vi "Point_Delete.vi"(8 "Error In":errorcluster, 10 "Tag":string, 11 "Map":T1) -> (0 "Error Out":errorcluster, 3 "Map Out":T1)   [LabVIEW 2017, in "PointValueMap.lvlib"]
doc: "Deletes a point from a map."
uses:
  <vilib>/addons/PointValueMap/PointValueMap.lvlib
  <vilib>/addons/PointValueMap/controls/PointMap.ctl
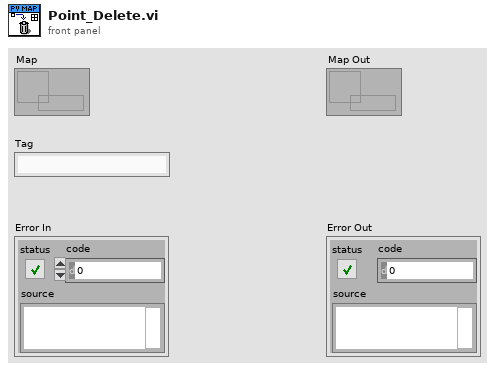
[diagram p1: front panel]
types:
  T1 = typedef "PointValueMap.lvlib/PointMap.ctl" = refnum<data-value>
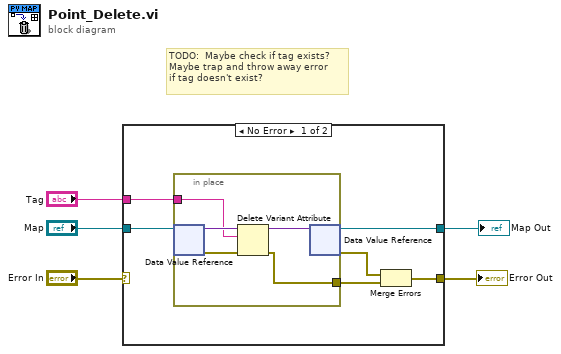
[diagram p0: block diagram]
diagram:
  # "TODO:  Maybe check if tag exists?\nMaybe trap and throw away error\nif tag doesn't exist?"
  n1 = case shown="No Error" "Error In" {
    selector: "Error In" -> [_ w18]
    tunnel: "Map" -> [w11 w17]
    tunnel: "Tag" -> [w10 _]
    tunnel: [w7 w18] -> w4
    tunnel: [w6 w17] -> w1
    frame No Error {
      n2 = in-place {
        in-place-border: w10 -> [w14]
        in-place-border: [w12] -> w8
        n3 = in-place-dvr #1(w11) -> (w16:variant, w15:errorcluster)
        n4 = Delete Variant Attribute(4:w15, 6:w14, 7:w16) -> (0:w12:errorcluster, 3:w13:variant)  [unwired: 1 out]
        n5 = in-place-dvr #1(w13) -> (w6:T1, w9:errorcluster)
      }
      n6 = Merge Errors(w9, w8) -> (w7:errorcluster)
    }
    frame Error {
    }
  }
  "Error Out" <- w4
  "Map Out" <- w1
